vi "test_VFH.vi"() -> ()   [LabVIEW 2019]
panel:
  out "Array":u16[][](array[numeric])=[[1, 2, 3, 4, 5, 6, 7, 8, 9, 10], [11, 12, 13, 14, 15, 16, 17, 18, 19, 20], [21, 200, 23, 24, 25, 26, 27, 28, 29, 30], [31, 32, 33, 34, 35, 36, 37, 38, 39, 40], [41, 42, 43, 44, 45, 46, 47, 48, 49, 50], [51, 52, 53, 54, 55, 56, 57, 58, 59, 60], [61, 62, 63, 64, 65, 66, 67, 68, 69, 70], [71, 72, 73, 74, 75, 76, 77, 78, 79, 80], [81, 82, 83, 84, 85, 86, 87, 200, 89, 90], [91, 92, 93, 94, 95, 96, 97, 98, 99, 100]]
  in  "end":cluster{"row":i32, "col":i32, "new val":u16}={"row"=8, "col"=7, "new val"=200}
  in  "start":cluster{"row":i32, "col":i32, "new val":u16}={"row"=2, "col"=1, "new val"=200}
  out "Intensity Graph":u16[][](graph)=[[1, 2, 3, 4, 5, 6, 7, 8, 9, 10], [11, 12, 13, 14, 15, 16, 17, 18, 19, 20], [21, 200, 23, 24, 25, 26, 27, 28, 29, 30], [31, 32, 33, 34, 35, 36, 37, 38, 39, 40], [41, 42, 43, 44, 45, 46, 47, 48, 49, 50], [51, 52, 53, 54, 55, 56, 57, 58, 59, 60], [61, 62, 63, 64, 65, 66, 67, 68, 69, 70], [71, 72, 73, 74, 75, 76, 77, 78, 79, 80], [81, 82, 83, 84, 85, 86, 87, 200, 89, 90], [91, 92, 93, 94, 95, 96, 97, 98, 99, 100]]
  in  "size":i32=10
  in  "element":u16=10
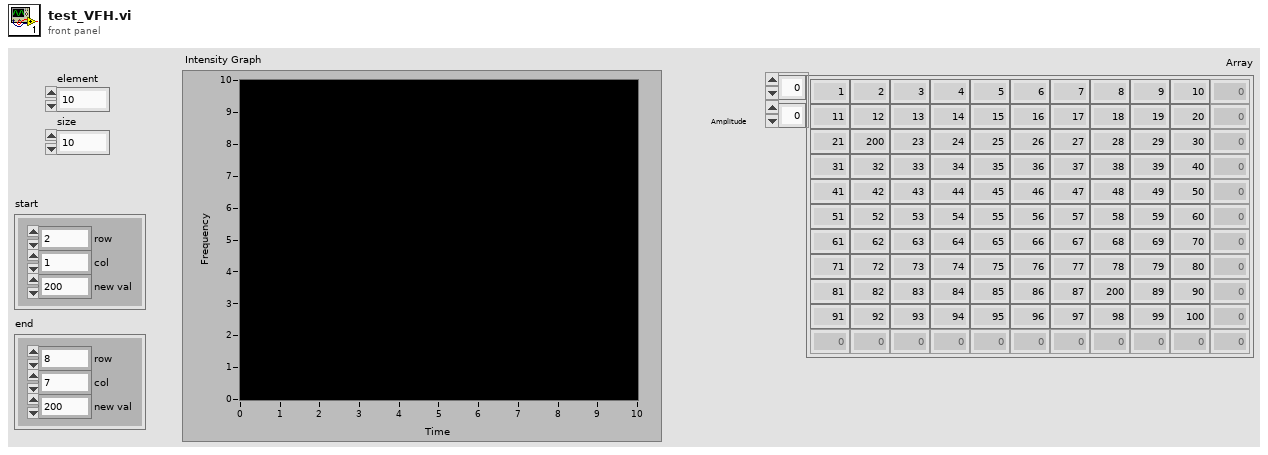
[diagram p1: front panel]
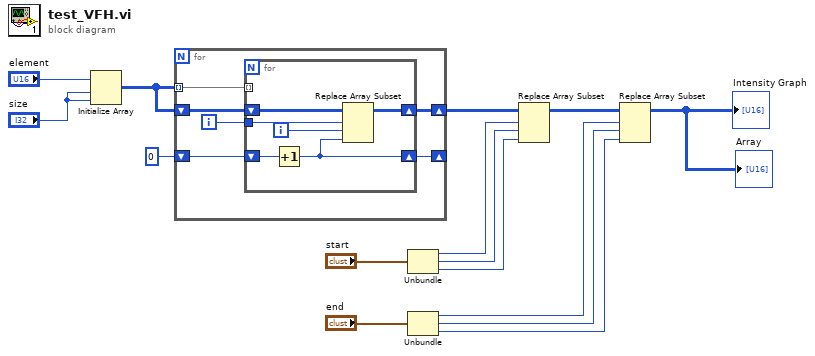
[diagram p0: block diagram]
diagram:
  n1 = Initialize Array("element", "size", "size") -> (w3:u16[][])
  n2 = for {
    shift-right: [w20] -> w2
    shift-left: w3 -> [w21]
    shift-right: [w17] -> _
    shift-left: 0 -> [w18]
    tunnel: w3 -> [w16] mode=indexing
    i -> [w19]
    n3 = for {
      shift-right: [w26] -> w20
      shift-left: w21 -> [w27]
      tunnel: w19 -> [w22]
      shift-right: [w24] -> w17
      shift-left: w18 -> [w25]
      tunnel: w16 -> [_] mode=indexing
      i -> [w23]
      n4 = Increment(x=w25) -> (x+1=w24:i32)
      n5 = Replace Array Subset(array=w27, new element=w24, index (row)=w22, index (col)=w23) -> (w26:u16[][])
    }
  }
  n6 = Unbundle("start") -> ("row"=w12:i32, "col"=w11:i32, "new val"=w10:u16)
  n7 = Unbundle("end") -> ("row"=w7:i32, "col"=w8:i32, "new val"=w9:u16)
  n8 = Replace Array Subset(array=w2, new element=w10, index (row)=w12, index (col)=w11) -> (w5:u16[][])
  n9 = Replace Array Subset(array=w5, new element=w9, index (row)=w7, index (col)=w8) -> (→"Intensity Graph" →"Array":u16[][])
